vi "读取生成OPF.vi"(8 "error in (no error)":errorcluster caption="错误输入（无错误）", 11 "EPUB输入":refnum<class "EPUB.lvclass">) -> (0 "error out":errorcluster caption="错误输出", 2 "OPF":string, 3 "EPUB输出":refnum<class "EPUB.lvclass">)   [LabVIEW 2016, in "EPUB.lvclass"]
uses:
  EPUB.lvclass
  EPUB.lvclass/EPUB.ctl
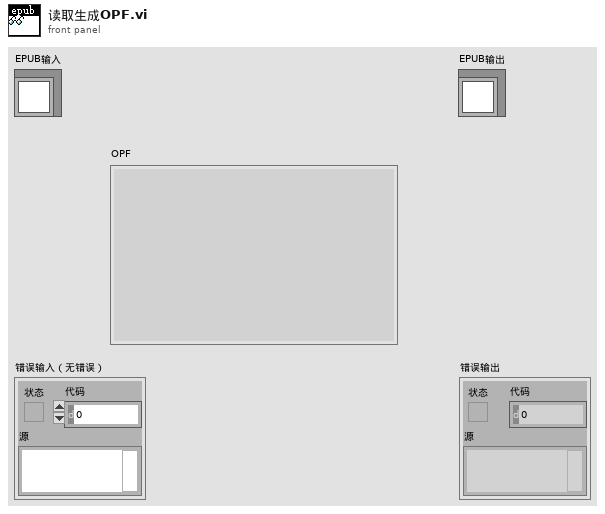
[diagram p1: front panel]
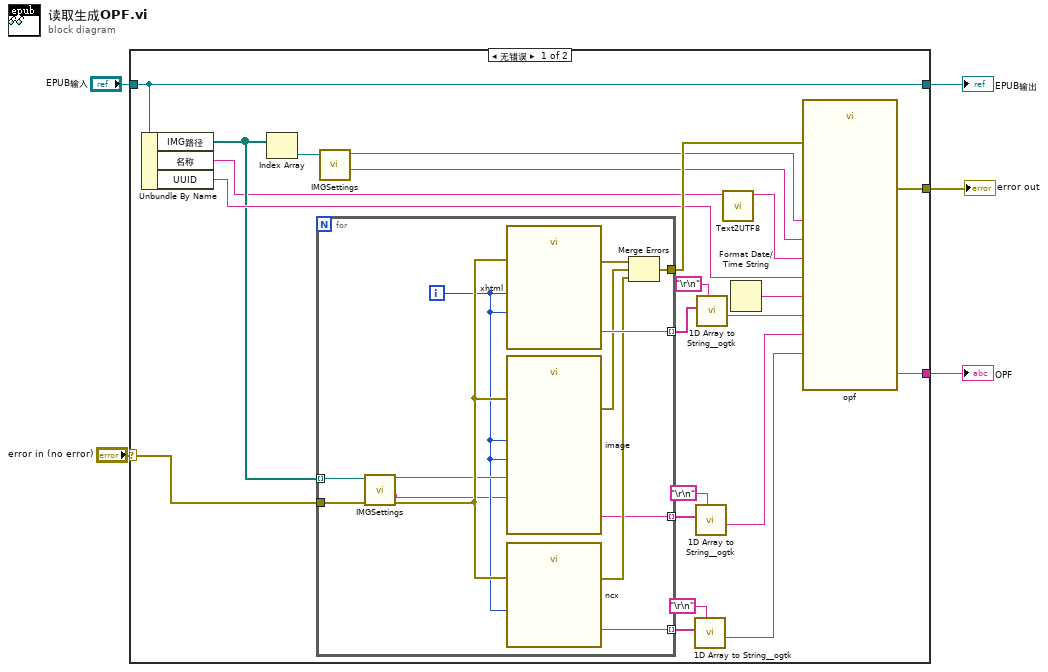
[diagram p0: block diagram]
diagram:
  n1 = case shown="无错误" "error in (no error)" {
    selector: "error in (no error)" -> [w26 w41]
    tunnel: [w18 w41] -> w4
    tunnel: [w27 w42] -> w2
    tunnel: "EPUB输入" -> [w27 w42]
    tunnel: [w17 _] -> w1
    frame No Error {
      n2 = Unbundle By Name(w27) -> ("IMG路径"=w11:path[], "名称"=w6:string, "UUID"=w12:string)
      n3 = Index Array(array=w11) -> (element=w9:path)  [unwired: 1 in]
      n4 = for {
        tunnel: w26 -> [w37]
        tunnel: [w40] -> w25 mode=indexing
        tunnel: [w29] -> w22 mode=indexing
        tunnel: [w39] -> w20 mode=indexing
        tunnel: w11 -> [w32] mode=indexing
        tunnel: [w33] -> w19
        i -> [w30]
        n5 = call "IMGSettings.vi"("error in (no error)"=w37, "IMG路径"=w32) -> ("error out"=w38:errorcluster, "type"=w28:string, "extension"=w31:string)  [unwired: 7 in]
        n6 = call "xhtml"("idx"=w30, "idx1"=w30, "error in (no error)"=w38) -> ("Result"=w40:string, "error out"=w36:errorcluster)  [unwired: 11 in]
        n7 = call "image"("imgTypt"=w28, "idx"=w30, "idx1"=w30, "extname"=w31, "error in (no error)"=w38) -> ("Result"=w29:string, "error out"=w35:errorcluster)  [unwired: 9 in]
        n8 = call "ncx"("idx"=w30, "error in (no error)"=w38) -> ("Result"=w39:string, "error out"=w34:errorcluster)  [unwired: 12 in]
        n9 = Merge Errors(w36, w35, w34) -> (w33:errorcluster)
      }
      n10 = call "IMGSettings.vi"("IMG路径"=w9) -> ("type"=w8:string, "extension"=w10:string)  [unwired: 8 in, 1 out]
      n11 = call <userlib>:"1D Array to String__ogtk.vi"("delimiter (Tab)"="\r\n", "Array of Strings"=w20) -> ("delimited string"=w13:string)  [unwired: 9 in]
      n12 = call <userlib>:"1D Array to String__ogtk.vi"("delimiter (Tab)"="\r\n", "Array of Strings"=w22) -> ("delimited string"=w14:string)  [unwired: 9 in]
      n13 = call <userlib>:"1D Array to String__ogtk.vi"("delimiter (Tab)"="\r\n", "Array of Strings"=w25) -> ("delimited string"=w15:string)  [unwired: 9 in]
      n14 = call <vilib>:"Text2UTF8.vi"("text"=w6) -> ("utf-8 text"=w7:string)  [unwired: 9 in, 1 out]
      n15 = Format Date/Time String() -> (date/time string=w16:string)  [unwired: 3 in]
      n16 = call "opf"("xhtml"=w15, "cover_type"=w8, "ncx"=w13, "title"=w7, "UUID"=w12, "date"=w16, "error in (no error)"=w19, "cover_ext"=w10, "img"=w14) -> ("Result"=w17:string, "error out"=w18:errorcluster)  [unwired: 5 in]
    }
    frame Error {
    }
  }
  "error out" <- w4
  "EPUB输出" <- w2
  "OPF" <- w1
